vi "processTaskRef.vi"(8 "error in (no error)":errorcluster, 11 "classPathToReplace":path) -> (0 "error out":errorcluster)   [LabVIEW 2023]
uses:
  <vilib>/Utility/traverseref.llb/TRef TravTarget.ctl
  <vilib>/Utility/traverseref.llb/VI Scripting - Traverse.lvlib
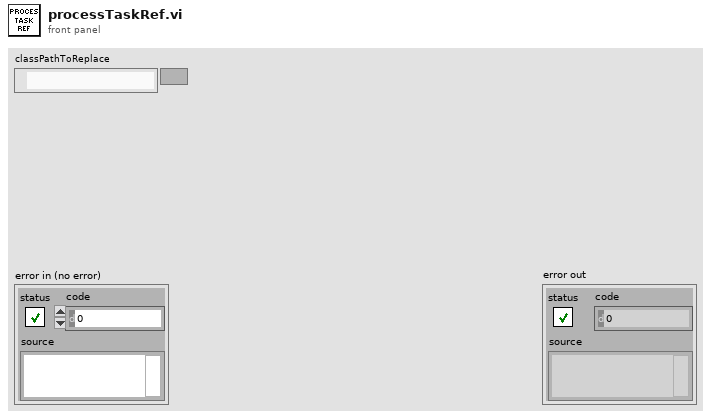
[diagram p1: front panel]
types:
  T1 = typedef "TRef TravTarget.ctl" = enum16{"FP", "BD", "Other"}
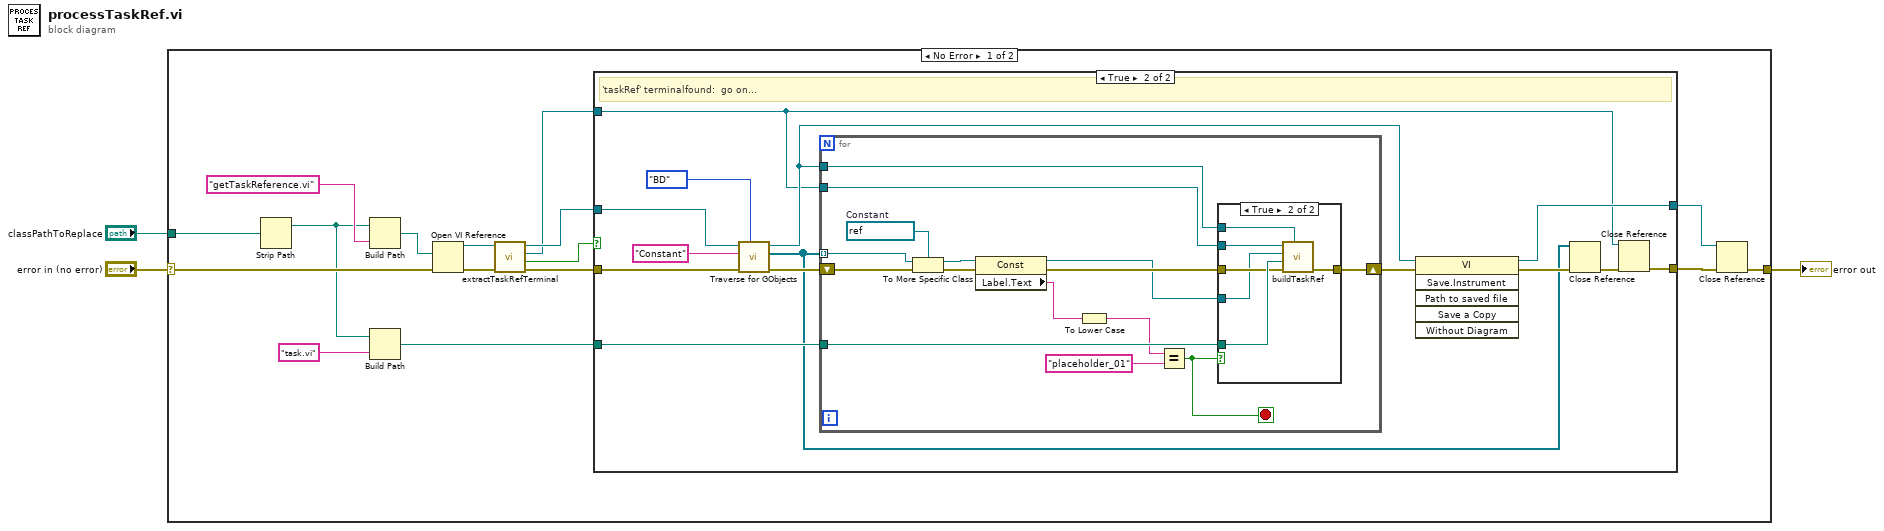
[diagram p0: block diagram]
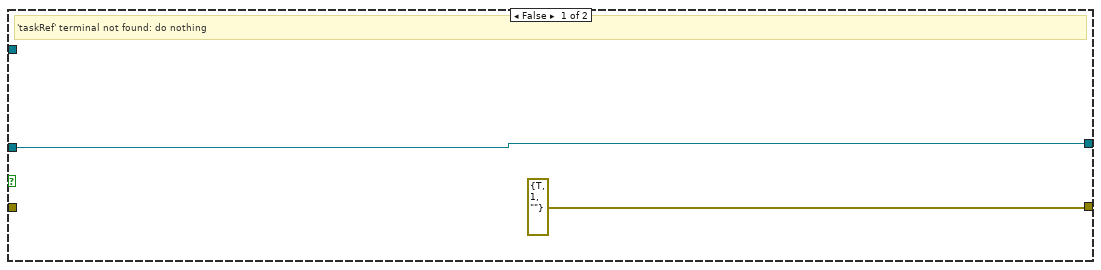
[diagram p2: hidden frame]
diagram:
  n1 = case shown="No Error" "error in (no error)" {
    selector: "error in (no error)" -> [w19 w58]
    tunnel: "classPathToReplace" -> [w14 _]
    tunnel: [w18 w58] -> w1
    frame No Error {
      n2 = Strip Path(path=w14) -> (stripped path=w11:path)  [unwired: 1 out]
      n3 = Build Path(base path=w11, name or relative path="getTaskReference.vi" ("String")) -> (appended path=w13:path)
      n4 = Build Path(base path=w11, name or relative path="task.vi" ("String")) -> (appended path=w10:path)
      n5 = Open VI Reference(vi path=w13, error in (no error)=w19) -> (vi reference=w8:refnum<vi>, error out=w9:errorcluster)  [unwired: 4 in]
      n6 = call "extractTaskRefTerminal.vi"("error in (no error)"=w9, "VI in"=w8) -> ("error out"=w6:errorcluster, "found?"=w5:bool, "taskRefTerminal"=w4:refnum<vi>, "VI out"=w7:refnum<vi>)  [unwired: 6 in]
      n7 = case shown="True" w5 {
        tunnel: [errorcluster {"status"=TRUE, "code"=1, "source"=""} ("error in") w26] -> w17
        tunnel: [w21 w35] -> w16
        tunnel: w10 -> [_ w33]
        tunnel: w7 -> [w21 w29]
        tunnel: w6 -> [_ w28]
        tunnel: w4 -> [_ w25]
        frame False {
          # "'taskRef' terminal not found: do nothing"
        }
        frame True {
          # "'taskRef' terminalfound:  go on..."
          n8 = call <vilib>:"Traverse for GObjects.vi"("Traverse Target"=TRef_TravTarget."BD", "error in (no error)"=w28, "Class Name"="Constant", "VI Refnum"=w29) -> ("error out"=w30:errorcluster, "References"=w22:refnum<vi>[], "dup VI Refnum"=w34:refnum<vi>)  [unwired: 4 in, 1 out]
          n9 = for {
            tunnel: w22 -> [w42] mode=indexing
            tunnel: w34 -> [w50]
            tunnel: w33 -> [w49]
            shift-right: [w39] -> w31
            shift-left: w30 -> [w38]
            tunnel: w25 -> [w37]
            stop <- w45 stop-if-true
            w41 = refnum<vi> refnum  # Constant
            n10 = To More Specific Class(target class=w41, reference=w42, error in=w38) -> (specific class reference=w43:refnum<vi>, error out=w44:errorcluster)
            n11 = property class="Const"(reference=w43, error in=w44) -> (reference out=w40:refnum<vi>, error out=w47:errorcluster, "Label.Text"=w48:string)
            n12 = To Lower Case(string=w48) -> (all lower case string=w46:string)
            n13 = Equal?(x=w46, y="placeholder_01" ("placeholderLabel")) -> (x = y?=w45:bool)
            n14 = case shown="True" w45 {
              tunnel: w50 -> [_ w57]
              tunnel: w49 -> [_ w56]
              tunnel: w47 -> [w51 w55]
              tunnel: w40 -> [_ w54]
              tunnel: [w51 w52] -> w39
              tunnel: w37 -> [_ w53]
              frame False {
              }
              frame True {
                n15 = call "buildTaskRef.vi"("targetVIRef"=w57, "error in (no error)"=w55, "taskPath"=w56, "Const Refnum"=w54, "taskRefTerminal"=w53) -> ("error out"=w52:errorcluster)  [unwired: 6 in]
              }
            }
          }
          n16 = invoke class="VI" method="Save.Instrument"(reference=w34, error in=w31) -> (reference out=w35:refnum<vi>, error out=w24:errorcluster)  [unwired: 4 in, 4 out]
          n17 = Close Reference(reference=w22, error in (no error)=w24) -> (error out=w23:errorcluster)
          n18 = Close Reference(reference=w25, error in (no error)=w23) -> (error out=w26:errorcluster)
        }
      }
      n19 = Close Reference(reference=w16, error in (no error)=w17) -> (error out=w18:errorcluster)
    }
    frame Error {
    }
  }
  "error out" <- w1
